vi "IOManipulating.vi"(8 "operation (0:open)":T1(ring), 11 "file path (use dialog)":path) -> (0 "Open Control 2":string[][](table), 3 "Table Control":string[][](table))   [LabVIEW 2023]
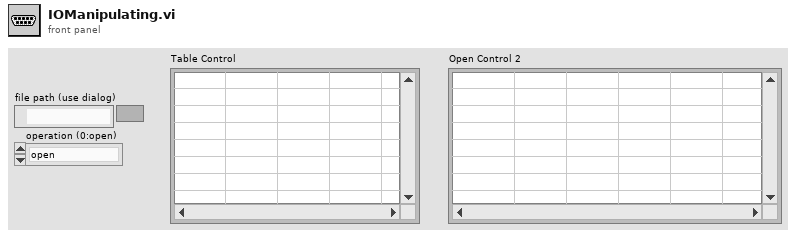
[diagram p1: front panel]
types:
  T1 = enum16{"open", "replace", "create", "open or create", "replace or create", "replace or create with confirmation"}
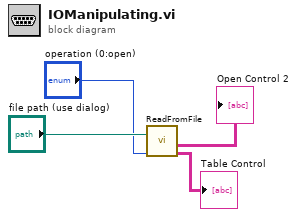
[diagram p0: block diagram]
diagram:
  n1 = call "ReadFromFile.vi"("operation (0:open)"="operation (0:open)", "file path (use dialog)"="file path (use dialog)") -> ("Open or create Control"=→"Table Control":string[][], "Open Control"=→"Open Control 2":string[][])  [unwired: 6 in, 2 out]
